vi "test-discretization-2.vi"() -> ()   [LabVIEW 2019]
uses:
  <vilib>/Analysis/Matrix/Datatypes/RealMatrix.ctl
  <vilib>/Analysis/baseanly.llb/Real A x B.vi
  <vilib>/Rock Robotics/WPI/ThirdParty/JAS_Junk/TrajLib/MatBuilder_Create.vi
  <vilib>/Analysis/7linalg.llb/Transpose Matrix.vi
  <vilib>/Analysis/7linalg.llb/Real Transpose Matrix.vi
  <vilib>/Rock Robotics/WPI/ThirdParty/JAS_Junk/TrajLib/MatrixHelper_CoerceSize.vi
  <vilib>/Rock Robotics/WPI/ThirdParty/JAS_Junk/TrajLib/Matrix_Ident.vi
  <vilib>/Analysis/Matrix/Numeric/Multiply/Multiply.vi
  <vilib>/Analysis/Matrix/Numeric/Multiply/Multiply - RM,R.vi
  <vilib>/Rock Robotics/WPI/ThirdParty/JAS_Junk/TrajLib/Matrix_Exp.vi
  <vilib>/Rock Robotics/WPI/ThirdParty/JAS_Junk/TrajLib/Matrix_AssignBlock.vi
  <vilib>/Rock Robotics/WPI/ThirdParty/JAS_Junk/TrajLib/Matrix_ExtractFrom.vi
  <vilib>/Analysis/7linalg.llb/Create Special Matrix.vi
  <vilib>/Analysis/7linalg.llb/Create Special Real Matrix.vi
  <vilib>/Analysis/Matrix/Numeric/Add/Add.vi
  <vilib>/Analysis/Matrix/Numeric/Add/Add - RM,RM.vi
  <vilib>/Rock Robotics/WPI/ThirdParty/JAS_Junk/TrajLib/Trajectory_Library.lvlib
  <vilib>/Analysis/NI_AALBase.lvlib
  <vilib>/Analysis/Matrix/NI_Matrix.lvlib
panel:
  out "Test Passed 2":bool
  out "Test Passed 1":bool
  out "Test Passed 0":bool
  out "AQ Err":bool
  out "AQ - DiscQ":T1
  out "AQ - DiscA":T1
  out "AB-Taylor-Err":bool
  out "ABTaylor-DiscB":T1
  out "ABTaylor - DiscA":T1
  out "AB-Err":bool
  out "AB-DiscB":T1
  out "AB - DiscA":T1
  out "x1-Disc":T1
  out "DiscA Error":bool
  out "DiscA":T1
  out "Cost Mat":T1
  out "CoVar Mat":T1
  # "1.0,   0.0,    0.0\n\n0.0,     4.0,   0.0, ;\n\n0.0,     0.0,  9.0;"
  # "1.0,      0.0,      0.0, \n\n0.0,   1.0 / 4.0,   0.0, \n\n0.0,       0.0,      1.0 / 9.0,"
  # "VecBuilder.fill(\n          x0.get(0, 0) + 1.0 * x0.get(1, 0), \n          x0.get(1, 0));"
  # "2,\n1"
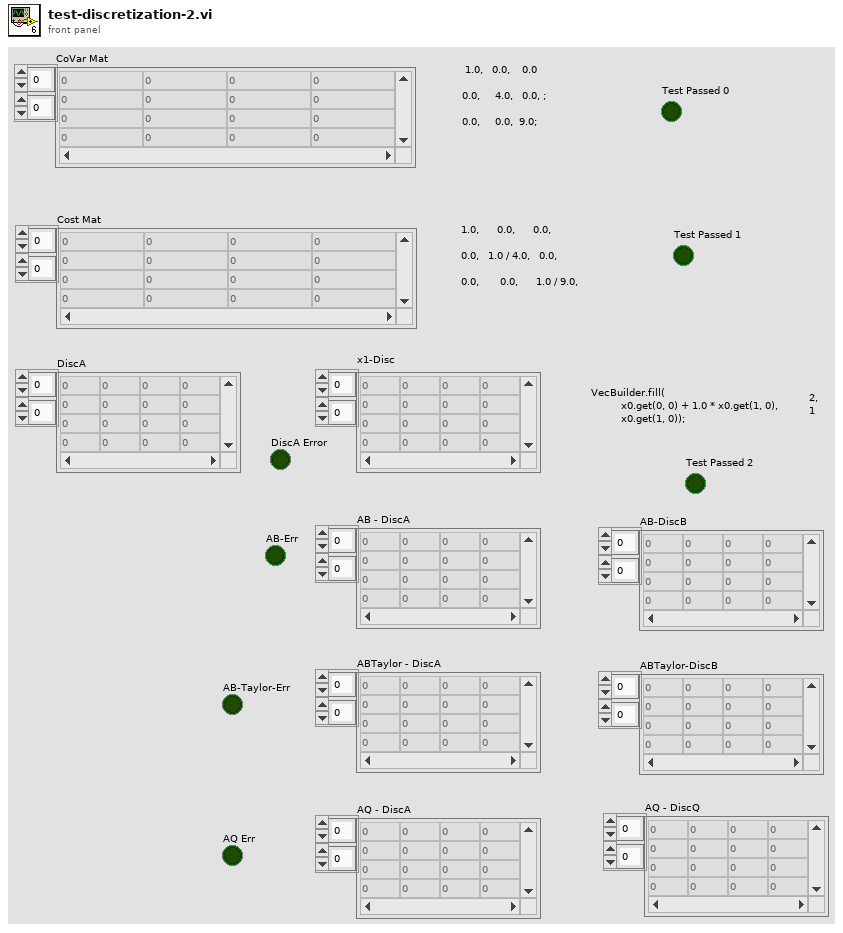
[diagram p1: front panel]
types:
  T1 = typedef "NI_Matrix.lvlib/RealMatrix.ctl" = dbl[][]
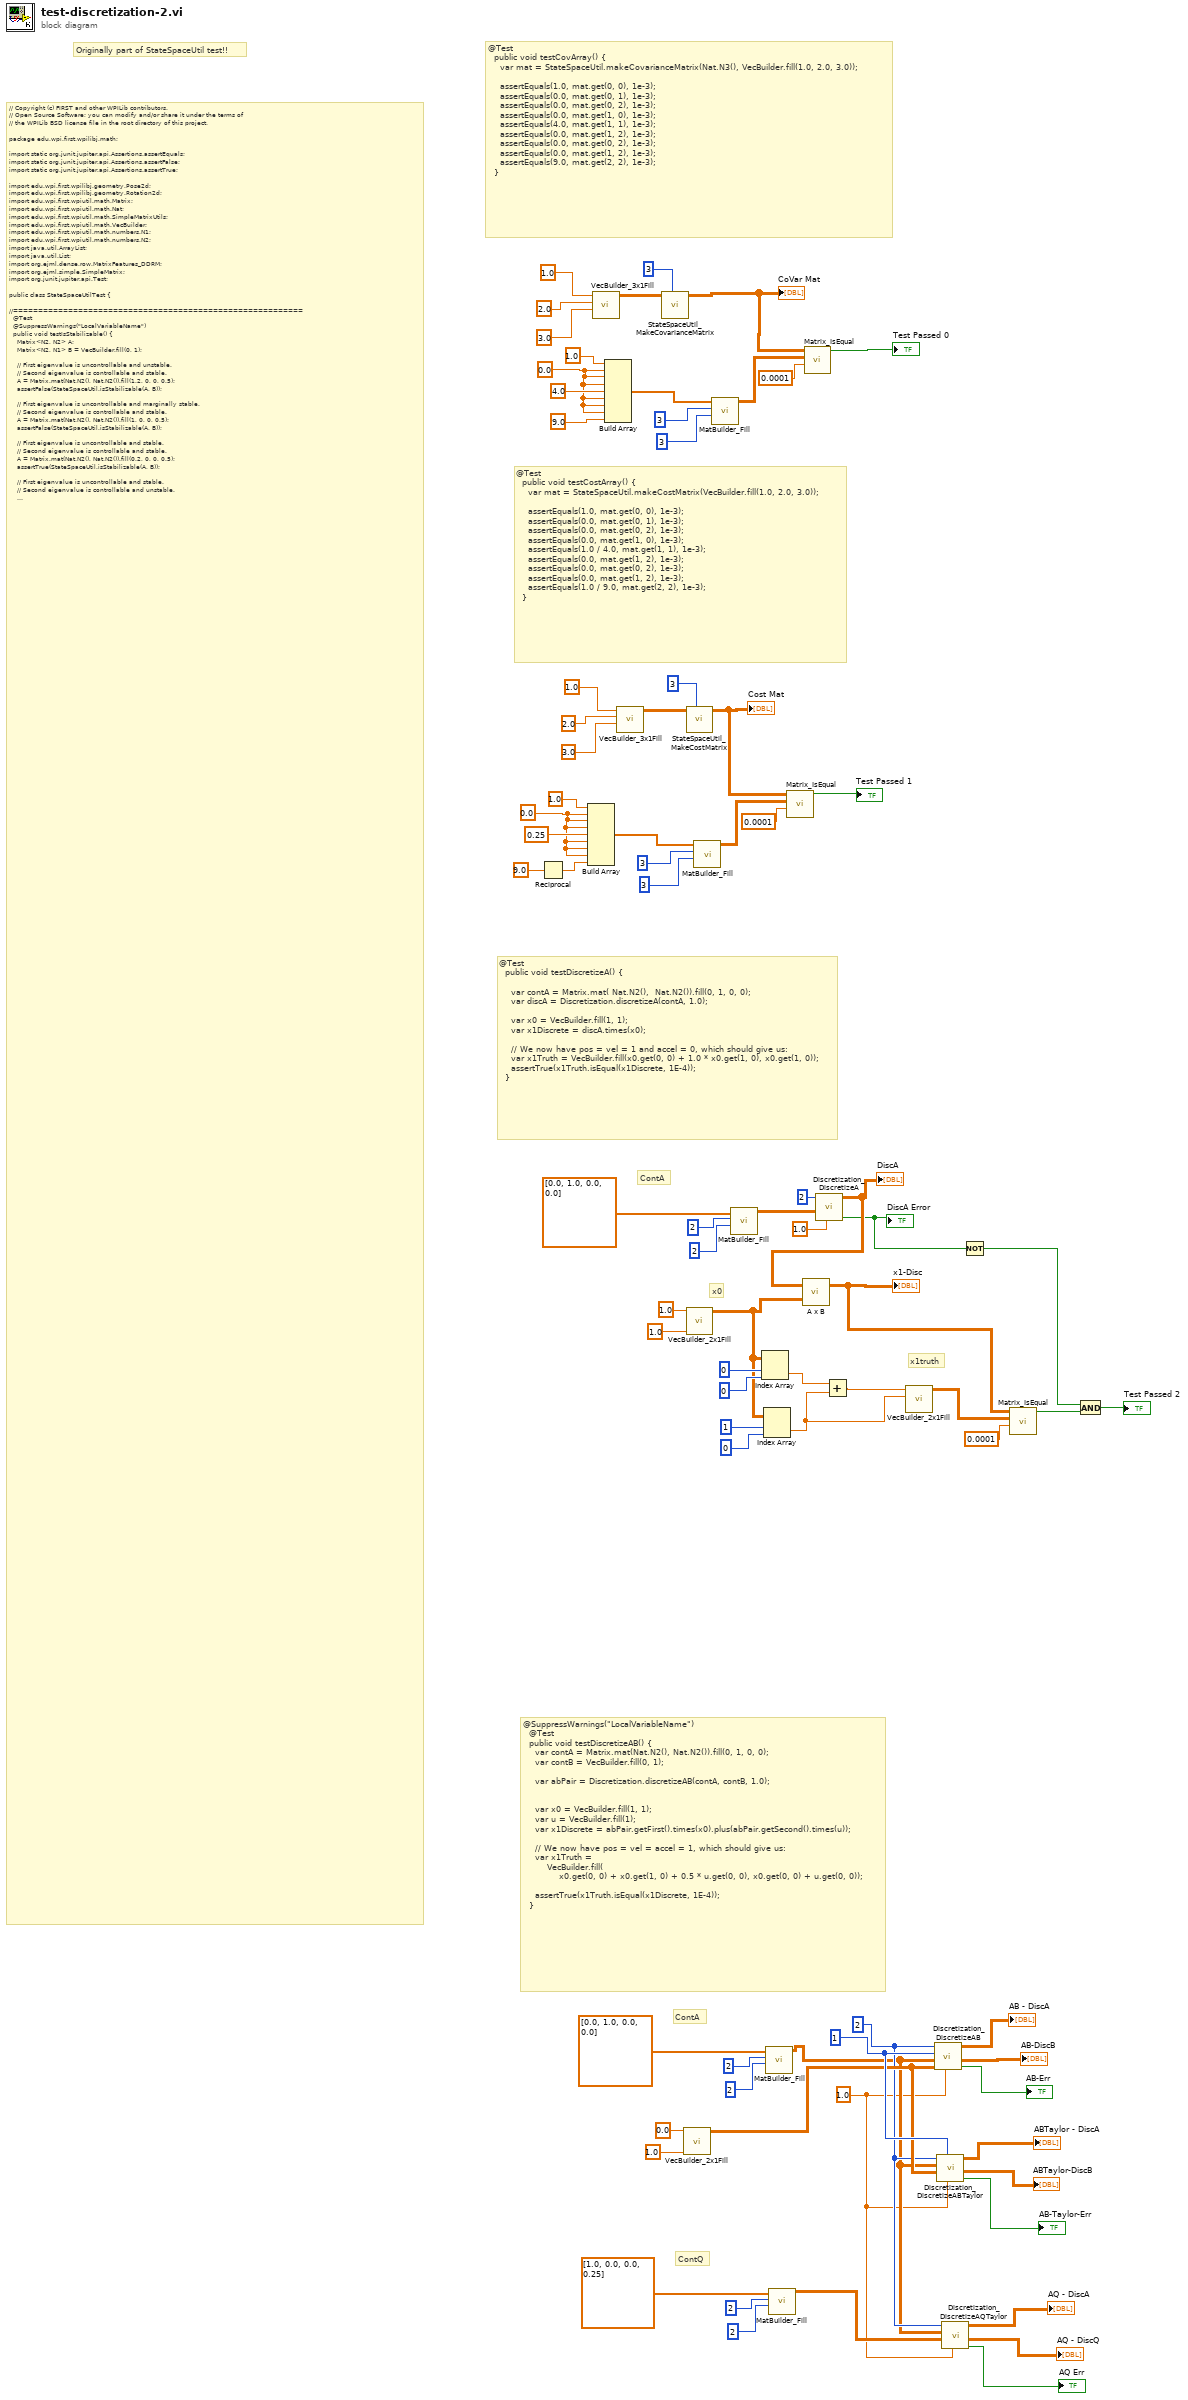
[diagram p0: block diagram]
diagram:
  w22 = 0.0 ("element")
  w33 = 0.0 ("element")
  w42 = 1.0 ("dT_Seconds")
  w56 = 1 ("Inputs")
  w45 = 2 ("States")
  # "x1truth"
  # "x0"
  # "Originally part of StateSpaceUtil test!!"
  # "ContQ"
  # "ContA"
  # "@SuppressWarnings(\"LocalVariableName\")\n  @Test\n  public void testDiscretizeAB() {\n    var contA = Matrix.mat(Nat.N2(), Nat.N2()).fill(0, 1, 0, 0);\n    var contB = VecBuilder.fill(0, 1);\n\n    var abPair = Discretization.discretizeAB(contA, contB, 1.0);\n\n\n    var x0 = VecBuilder.fill(1, 1);\n    var u = VecBuilder.fill(1);\n    var x1Discrete = abPair.getFirst().times(x0).plus(abPair.getSecond().times(u));\n\n    // We now have pos = vel = accel = 1, which should give us:\n    var x1Truth =\n        VecBuilder.fill(\n            x0.get(0, 0) + x0.get(1, 0) + 0.5 * u.get(0, 0), x0.get(0, 0) + u.get(0, 0));\n\n    assertTrue(x1Truth.isEqual(x1Discrete, 1E-4));\n  }"
  # "ContA"
  # "@Test\n  public void testDiscretizeA() {\n\n    var contA = Matrix.mat( Nat.N2(),  Nat.N2()).fill(0, 1, 0, 0);\n    var discA = Discretization.discretizeA(contA, 1.0);\n\n    var x0 = VecBuilder.fill(1, 1);\n    var x1Discrete = discA.times(x0);\n\n    // We now have pos = vel = 1 and accel = 0, which should give us:\n    var x1Truth = VecBuilder.fill(x0.get(0, 0) + 1.0 * x0.get(1, 0), x0.get(1, 0));\n    assertTrue(x1Truth.isEqual(x1Discrete, 1E-4));\n  }"
  # "@Test\n  public void testCostArray() {\n    var mat = StateSpaceUtil.makeCostMatrix(VecBuilder.fill(1.0, 2.0, 3.0));\n\n    assertEquals(1.0, mat.get(0, 0), 1e-3);\n    assertEquals(0.0, mat.get(0, 1), 1e-3);\n    assertEquals(0.0, mat.get(0, 2), 1e-3);\n    assertEquals(0.0, mat.get(1, 0), 1e-3);\n    assertEquals(1.0 / 4.0, mat.get(1, 1), 1e-3);\n    assertEquals(0.0, mat.get(1, 2), 1e-3);\n    assertEquals(0.0, mat.get(0, 2), 1e-3);\n    assertEquals(0.0, mat.get(1, 2), 1e-3);\n    assertEquals(1.0 / 9.0, mat.get(2, 2), 1e-3);\n  }"
  # "@Test\n  public void testCovArray() {\n    var mat = StateSpaceUtil.makeCovarianceMatrix(Nat.N3(), VecBuilder.fill(1.0, 2.0, 3.0));\n\n    assertEquals(1.0, mat.get(0, 0), 1e-3);\n    assertEquals(0.0, mat.get(0, 1), 1e-3);\n    assertEquals(0.0, mat.get(0, 2), 1e-3);\n    assertEquals(0.0, mat.get(1, 0), 1e-3);\n    assertEquals(4.0, mat.get(1, 1), 1e-3);\n    assertEquals(0.0, mat.get(1, 2), 1e-3);\n    assertEquals(0.0, mat.get(0, 2), 1e-3);\n    assertEquals(0.0, mat.get(1, 2), 1e-3);\n    assertEquals(9.0, mat.get(2, 2), 1e-3);\n  }"
  # "// Copyright (c) FIRST and other WPILib contributors.\n// Open Source Software; you can modify and/or share it under the terms of\n// the WPILib BSD license file in the root directory of this project.\n\npackage edu.wpi.first.wpilibj.math;\n\nimport static org.junit.jupiter.api.Assertions.assertEquals;\nimport static org.junit.jupiter.api.Assertions.assertFalse;\nimport static org.junit.jupiter.api.Assertions.assertTrue;\n\nimport edu.wpi.first.wpilibj.geometry.Pose2d;\nimport edu.wpi.first.wpilibj.geometry.Rotation2d;\nimport edu.wpi.first.wpiutil.math.Matrix;\nimport edu.wpi.first.wpiutil.math.Nat;\nimport edu.wpi.first.wpiutil.math.SimpleMatrixUtils;\nimport edu.wpi.first.wpiutil.math.VecBuilder;\nimport edu.wpi.first.wpiutil.math.numbers.N1;\nimport edu.wpi.first.wpiutil.math.numbers.N2;\nimport java.util.ArrayList;\nimport java.util.List;\nimport org.ejml.dense.row.MatrixFeatures_DDRM;\nimport org.ejml.simple.SimpleMatrix;\nimport org.junit.jupiter.api.Test;\n\npublic class StateSpaceUtilTest {\n\n//==========================================================\n  @Test\n  @SuppressWarnings(\"LocalVariableName\")\n  public void testIsStabilizable() {\n    Matrix<N2, N2> A;\n    Matrix<N2, N1> B = VecBuilder.fill(0, 1);\n\n    // First eigenvalue is uncontrollable and unstable.\n    // Second eigenvalue is controllable and stable.\n    A = Matrix.mat(Nat.N2(), Nat.N2()).fill(1.2, 0, 0, 0.5);\n    assertFalse(StateSpaceUtil.isStabilizable(A, B));\n\n    // First eigenvalue is uncontrollable and marginally stable.\n    // Second eigenvalue is controllable and stable.\n    A = Matrix.mat(Nat.N2(), Nat.N2()).fill(1, 0, 0, 0.5);\n    assertFalse(StateSpaceUtil.isStabilizable(A, B));\n\n    // First eigenvalue is uncontrollable and stable.\n    // Second eigenvalue is controllable and stable.\n    A = Matrix.mat(Nat.N2(), Nat.N2()).fill(0.2, 0, 0, 0.5);\n    assertTrue(StateSpaceUtil.isStabilizable(A, B));\n\n    // First eigenvalue is uncontrollable and stable.\n    // Second eigenvalue is controllable and unstable.\n    A = Matrix.mat(Nat.N2(), Nat.N2()).fill(0.2, 0, 0, 1.2);\n    assertTrue(StateSpaceUtil.isStabilizable(A, B));\n  }\n\n//==========================================================\n  @Test\n  public void testMakeWhiteNoiseVector() {\n    var firstData = new ArrayList<Double>();\n    var secondData = new ArrayList<Double>();\n    for (int i = 0; i < 1000; i++) {\n      var noiseVec = StateSpaceUtil.makeWhiteNoiseVector(VecBuilder.fill(1.0, 2.0));\n      firstData.add(noiseVec.get(0, 0));\n      secondData.add(noiseVec.get(1, 0));\n    }\n    assertEquals(1.0, calculateStandardDeviation(firstData), 0.2);\n    assertEquals(2.0, calculateStandardDeviation(secondData), 0.2);\n  }\n\n  private double calculateStandardDeviation(List<Double> numArray) {\n    double sum = 0.0;\n    double standardDeviation = 0.0;\n    int length = numArray.size();\n\n    for (double num : numArray) {\n      sum += num;\n    }\n\n    double mean = sum / length;\n\n    for (double num : numArray) {\n      standardDeviation += Math.pow(num - mean, 2);\n    }\n\n    return Math.sqrt(standardDeviation / length);\n  }\n\n\n//==========================================================\n    @Test\n  public void testMatrixExp() {\n    Matrix<N2, N2> wrappedMatrix = Matrix.eye(Nat.N2());\n    var wrappedResult = wrappedMatrix.exp();\n\n    assertTrue(\n        wrappedResult.isEqual(Matrix.mat(Nat.N2(), Nat.N2()).fill(Math.E, 0, 0, Math.E), 1E-9));\n\n    var matrix = Matrix.mat(Nat.N2(), Nat.N2()).fill(1, 2, 3, 4);\n    wrappedResult = matrix.times(0.01).exp();\n\n    assertTrue(\n        wrappedResult.isEqual(\n            Matrix.mat(Nat.N2(), Nat.N2()).fill(1.01035625, 0.02050912, 0.03076368, 1.04111993),\n            1E-8));\n  }\n\n//==========================================================\n  @Test\n  public void testSimpleMatrixExp() {\n    SimpleMatrix matrix = SimpleMatrixUtils.eye(2);\n    var result = SimpleMatrixUtils.exp(matrix);\n\n    assertTrue(\n        MatrixFeatures_DDRM.isIdentical(\n            result.getDDRM(),\n            new SimpleMatrix(2, 2, true, new double[] {Math.E, 0, 0, Math.E}).getDDRM(),\n            1E-9));\n\n    matrix = new SimpleMatrix(2, 2, true, new double[] {1, 2, 3, 4});\n    result = SimpleMatrixUtils.exp(matrix.scale(0.01));\n\n    assertTrue(\n        MatrixFeatures_DDRM.isIdentical(\n            result.getDDRM(),\n            new SimpleMatrix(\n                    2, 2, true, new double[] {1.01035625, 0.02050912, 0.03076368, 1.04111993})\n                .getDDRM(),\n            1E-8));\n  }\n\n//==========================================================\n  @Test\n  public void testPoseToVector() {\n    Pose2d pose = new Pose2d(1, 2, new Rotation2d(3));\n    var vector = StateSpaceUtil.poseToVector(pose);\n    assertEquals(pose.getTranslation().getX(), vector.get(0, 0), 1e-6);\n    assertEquals(pose.getTranslation().getY(), vector.get(1, 0), 1e-6);\n    assertEquals(pose.getRotation().getRadians(), vector.get(2, 0), 1e-6);\n  }\n}"
  n1 = Reciprocal(x=9.0 ("element")) -> (1/x=w18:dbl)
  n2 = Build Array(1.0 ("element"), w22, w22, w22, 0.25 ("element"), w22, w22, w22, w18) -> (w25:dbl[])
  n3 = call <vilib>:"VecBuilder_3x1Fill.vi"("R2"=3.0, "R1"=2.0, "R0"=1.0) -> ("output matrix"=w77:T1)  [unwired: 8 in]
  n4 = Build Array(1.0 ("element"), w33, w33, w33, 4.0 ("element"), w33, w33, w33, 9.0 ("element")) -> (w36:dbl[])
  n5 = call <vilib>:"VecBuilder_3x1Fill.vi"("R2"=3.0, "R1"=2.0, "R0"=1.0) -> ("output matrix"=w72:T1)  [unwired: 8 in]
  n6 = call <vilib>:"StateSpaceUtil_MakeCovarianceMatrix.vi"("States"=3, "StdDevs"=w77) -> ("Covariance Matrix"=w31:T1)  [unwired: 8 in, 1 out]
  "CoVar Mat" <- w31
  n7 = call <vilib>:"VecBuilder_2x1Fill.vi"("R1"=1.0, "R0"=0.0 ("R0_C0")) -> ("output matrix"=w55:T1)  [unwired: 9 in]
  n8 = call <vilib>:"StateSpaceUtil_MakeCostMatrix.vi"("States"=3, "Costs"=w72) -> ("Costs Matrix"=w17:T1)  [unwired: 8 in, 1 out]
  "Cost Mat" <- w17
  n9 = call <vilib>:"VecBuilder_2x1Fill.vi"("R1"=1.0, "R0"=1.0 ("R0_C0")) -> ("output matrix"=w10:T1)  [unwired: 9 in]
  n10 = call <vilib>:"MatBuilder_Fill.vi"("Columns"=3, "Rows"=3, "Value List"=w25) -> ("output matrix"=w21:T1)  [unwired: 6 in, 2 out]
  n11 = call <vilib>:"MatBuilder_Fill.vi"("Columns"=3, "Rows"=3, "Value List"=w36) -> ("output matrix"=w30:T1)  [unwired: 6 in, 2 out]
  n12 = call <vilib>:"MatBuilder_Fill.vi"("Columns"=2, "Rows"=2, "Value List"=dbl[] [0.0, 1.0, 0.0, 0.0]) -> ("output matrix"=w65:T1)  [unwired: 6 in, 2 out]
  n13 = Index Array(array=w10, index (row)=0, index (col)=0) -> (element=w9:dbl)
  n14 = Index Array(array=w10, index (row)=1, index (col)=0) -> (element=w7:dbl)
  n15 = call <vilib>:"MatBuilder_Fill.vi"("Columns"=2, "Rows"=2, "Value List"=dbl[] [0.0, 1.0, 0.0, 0.0]) -> ("output matrix"=w44:T1)  [unwired: 6 in, 2 out]
  n16 = call <vilib>:"MatBuilder_Fill.vi"("Columns"=2, "Rows"=2, "Value List"=dbl[] [1.0, 0.0, 0.0, 0.25]) -> ("output matrix"=w43:T1)  [unwired: 6 in, 2 out]
  n17 = call <vilib>:"Matrix_IsEqual.vi"("Tolerance"=0.0001, "other"=w21, "input matrix"=w17) -> ("Equal"=→"Test Passed 1":bool)  [unwired: 8 in]
  n18 = call <vilib>:"Matrix_IsEqual.vi"("Tolerance"=0.0001, "other"=w30, "input matrix"=w31) -> ("Equal"=→"Test Passed 0":bool)  [unwired: 8 in]
  n19 = call <vilib>:"Discretization_DiscretizeA.vi"("dT_Seconds"=1.0, "ContA"=w65, "States"=2) -> ("Error"=w2:bool, "DiscA"=w62:T1)  [unwired: 7 in]
  "DiscA" <- w62
  "DiscA Error" <- w2
  n20 = call-poly <vilib>:"A x B.vi"("B"=w10, "A"=w62) -> ("A x B"=w6:T1)  [unwired: 1 out]
  "x1-Disc" <- w6
  n21 = Add(x=w9, y=w7) -> (x+y=w8:dbl)
  n22 = call <vilib>:"VecBuilder_2x1Fill.vi"("R1"=w7, "R0"=w8) -> ("output matrix"=w5:T1)  [unwired: 9 in]
  n23 = call <vilib>:"Discretization_DiscretizeAB.vi"("dT_Seconds"=w42, "ContB"=w55, "ContA"=w44, "Inputs"=w56, "States"=w45) -> ("Error"=→"AB-Err":bool, "DiscB"=→"AB-DiscB":T1, "DiscA"=→"AB - DiscA":T1)  [unwired: 4 in]
  n24 = call <vilib>:"Discretization_DiscretizeABTaylor.vi"("dT_Seconds"=w42, "Inputs"=w56, "ContB"=w55, "ContA"=w44, "States"=w45) -> ("Error"=→"AB-Taylor-Err":bool, "DiscB"=→"ABTaylor-DiscB":T1, "DiscA"=→"ABTaylor - DiscA":T1)  [unwired: 4 in]
  n25 = call <vilib>:"Discretization_DiscretizeAQTaylor.vi"("dT_Seconds"=w42, "ContQ"=w43, "ContA"=w44, "States"=w45) -> ("Error"=→"AQ Err":bool, "DiscQ"=→"AQ - DiscQ":T1, "DiscA"=→"AQ - DiscA":T1)  [unwired: 5 in]
  n26 = Not(x=w2) -> (.not. x?=w1:bool)
  n27 = call <vilib>:"Matrix_IsEqual.vi"("Tolerance"=0.0001, "other"=w5, "input matrix"=w6) -> ("Equal"=w3:bool)  [unwired: 8 in]
  n28 = Compound Arithmetic op=AND(w1, w3) -> (→"Test Passed 2":bool)
